vi "GetObjectStatus.vi"(0 "reference in":refnum<class "G#Interface.lvclass">, 2 "simple info (F)":bool, 5 "error in (no error)":errorcluster) -> (8 "full class name":string, 9 "# of users":i32, 10 "all object names":string[](array[string]), 11 "last user?":bool, 12 "# of objects":i32, 13 "class name":string, 14 "reference out":refnum<class "G#Interface.lvclass">, 15 "not a refnum?":bool, 16 "object name":string, 17 "all refs out":refnum<class "G#Object.lvclass">[](array[class]), 18 "counter?":bool, 19 "error out":errorcluster)   [LabVIEW 2020, in "G#Interface.lvclass"]
doc: "Returns information about the specified object. If simple info = true, only object info is return and not the arrays of objects.\n\nIf input reference is unwired, only information about the class is returned."
uses:
  <vilib>/addons/_AddQ/G#Interface/G#Interface.lvclass
  <vilib>/addons/_AddQ/G#Object/G#Object.lvclass
  <vilib>/addons/_AddQ/G#Interface/G#Interface.lvclass/G#Interface.ctl
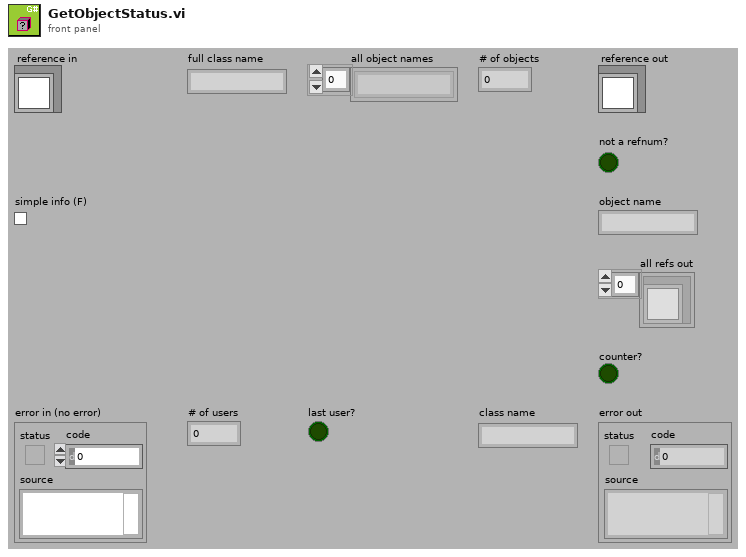
[diagram p1: front panel]
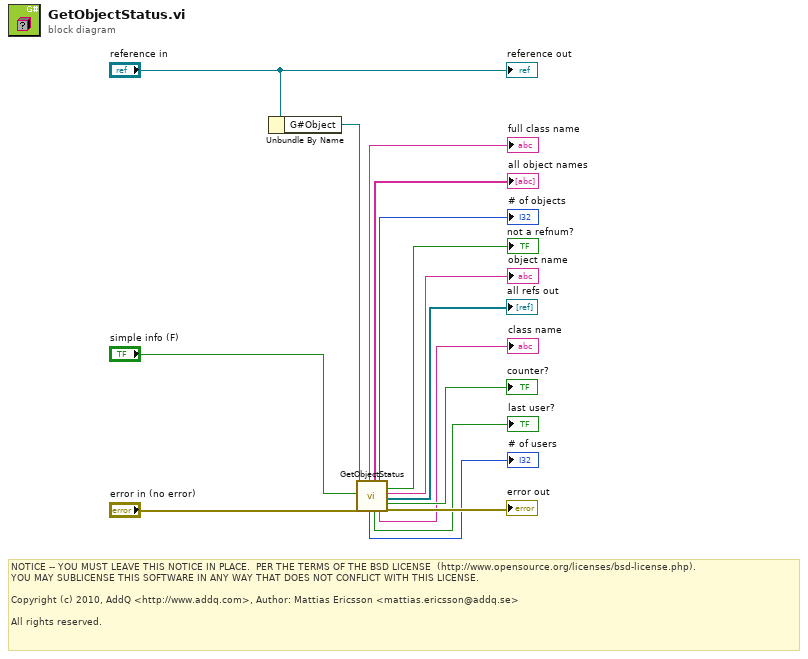
[diagram p0: block diagram]
diagram:
  # "NOTICE -- YOU MUST LEAVE THIS NOTICE IN PLACE.  PER THE TERMS OF THE BSD LICENSE  (http://www.opensource.org/licenses/bsd-license.php).\nYOU MAY SUBLICENSE THIS SOFTWARE IN ANY WAY THAT DOES NOT CONFLICT WITH THIS LICENSE.\n\nCopyright (c) 2010, AddQ <http://www.addq.com>, Author: Mattias Ericsson <mattias.ericsson@addq.se>\n\nAll rights reserved."
  n1 = Unbundle By Name("reference in") -> ("G#Object"=w13:refnum<class "G#Object.lvclass">)
  n2 = call-dynamic "GetObjectStatus.vi"("reference in"=w13, "simple info (F)"="simple info (F)", "error in (no error)"="error in (no error)") -> ("full class name"=→"full class name":string, "# of users?"=→"# of users":i32, "all object names"=→"all object names":string[], "last user"=→"last user?":bool, "# of objects"=→"# of objects":i32, "class name"=→"class name":string, "not a refnum?"=→"not a refnum?":bool, "object name"=→"object name":string, "all refs out"=→"all refs out":refnum<class "G#Object.lvclass">[], "counter?"=→"counter?":bool, "error out"=→"error out":errorcluster)  [unwired: 5 in, 1 out]
  "reference out" <- "reference in"
